vi "cam_wheel.vi"(7 "에러 입력":errorcluster, 10 "FPGA VI 참조 입력":refnum<k20>) -> (0 "에러 출력":errorcluster, 1 "거리":dbl, 2 "차체각도":dbl=-36.05, 3 "FPGA VI 참조 출력":refnum<k20>)   [LabVIEW 2019]
uses:
  <vilib>/Platform/TimedLoop/XDataNode/timing_clust.ctl
  <vilib>/Platform/TimedLoop/XDataNode/nitl_modes.ctl
  <vilib>/Platform/TimedLoop/XDataNode/wakeup.ctl
  <vilib>/myRIO/Instrument Drivers/Onboard IO/UART/typedef/VISA Configuration.ctl
  <vilib>/Utility/error.llb/Error Cluster From Error Code.vi
  <vilib>/rvi/errors/niLvFpgaAdjustHostInterfaceError.vi
  <vilib>/rvi/interface/nirviReadWriteControl/nirviReadWriteControl.xnode
  <vilib>/Platform/TimedLoop/XDataNode/XDataNode.xnode
  <vilib>/Platform/TimedLoop/XDataNode/XDNodeRunTimeDep.lvlib
  <vilib>/rvi/interface/Simulation/niFpgaSimulationCallBeginRW.vi
  NiFpgaLv.dll
  <vilib>/myRIO/Instrument Drivers/Onboard IO/UART/UART.lvlib
panel:
  out "pwm":dbl
  out "카메라 불인식 Y/N":bool
  in  "timed 정지":bool
  in  "Left":dbl[](array[numeric])=[2800.0, -379.347, 8600.0]
  in  "Right":dbl[](array[numeric])=[2800.0, 290.0, 8600.0]
  out "2번(불까지거리)":string
  out "1번(x픽셀)":string
  out "회전수 i":i32=148
  out "타임아웃":i32=-1
  out "L_encoder":i32
  out "R_Encoder":i32
  out "L_이동 거리":dbl=7.9770497222561305
  out "R_이동 거리":dbl=2.830566030477983
  out "mm/ms":dbl
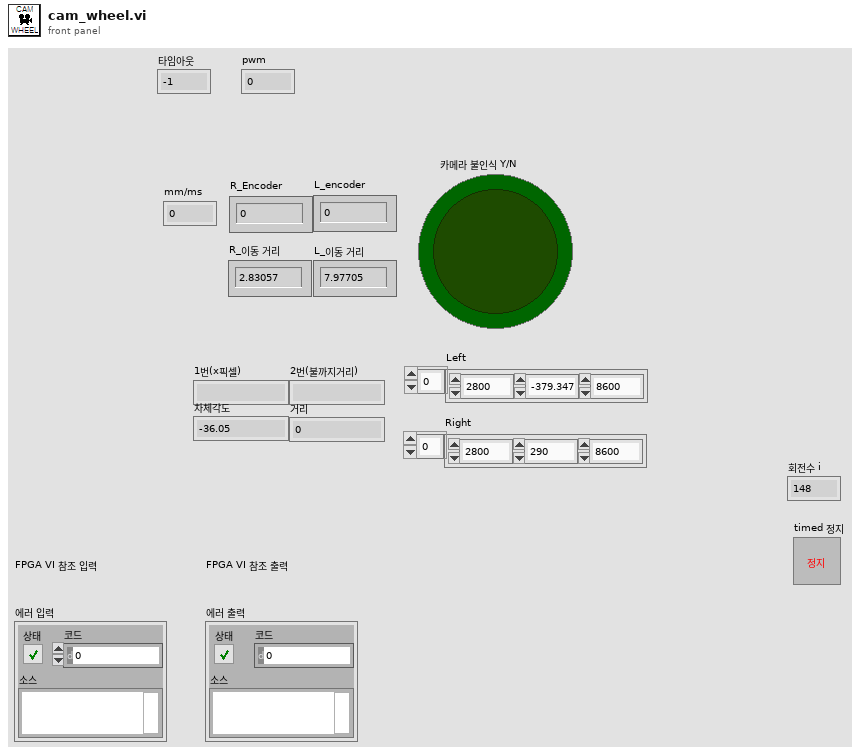
[diagram p1: front panel]
types:
  T1 = typedef "XDNodeRunTimeDep.lvlib/timing_clust.ctl" = cluster{"Expected End [f-1]":u64, "Actual End [f-1]":u64, "Finished Late? [f-1]":bool, "Expected End [i-1]":u64, "Actual End [i-1]":u64, "Finished Late? [i-1]":bool, "Expected Start [i]":u64, "Actual Start [i]":u64, "Expected Start [f]":u64, "Actual Start [f]":u64, "Source Name":string, "Structure Name":string, "Period":i64, "Deadline":i64, "Offset":i64, "Start":i64, "Priority":i32, "Timeout":i32, "Mode":T2, "Wakeup Reason":T3, "Error":errorcluster, "Source Type":string, "Secondary Source Type":string, "Global End Time":u64, "Global Start Time":u64, "Frame Duration":u64, "Iteration Duration":u64, "Assigned CPU":i32, "I/O Scan Engine Mode":u32}
  T2 = typedef "XDNodeRunTimeDep.lvlib/nitl_modes.ctl" = enum32{"No Change", "Process missed periods, maintain original phase", "Discard missed periods, maintain original phase", "Process missed periods, ignore original phase", "Discard missed periods, ignore original phase"}
  T3 = typedef "XDNodeRunTimeDep.lvlib/wakeup.ctl" = enum32{"Normal", "Aborted", "Asynchronous wakeup", "Timing source error", "Timed loop error", "Timeout"}
  T4 = typedef "UART.lvlib/VISA Configuration.ctl" = cluster{"baud rate (9600)":u32, "data bits (8)":u16, "parity (0:none)":enum16{"None", "Odd", "Even", "Mark", "Space"}, "stop bits (10: 1 bit)":u16, "flow control (0:none)":u16, "termination char\n(0xA = '\\n' = LF) ":u8, "Enable Termination\nChar (T)":bool, "timeout (10sec)":u32}
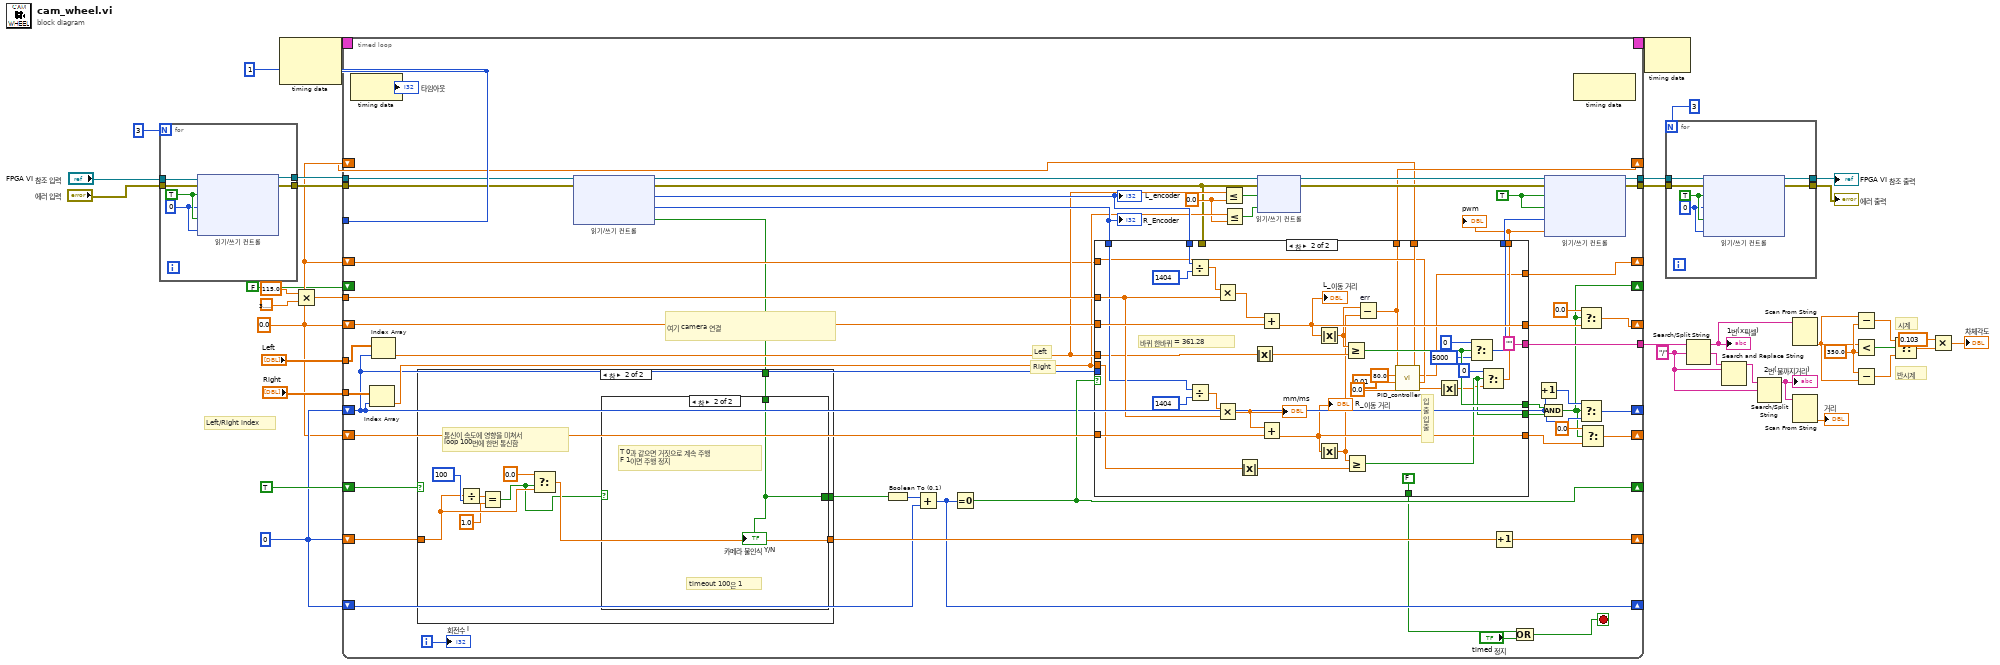
[diagram p0: block diagram]
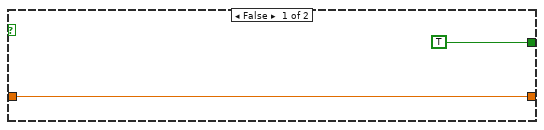
[diagram p2: hidden frame]
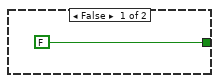
[diagram p3: hidden frame]
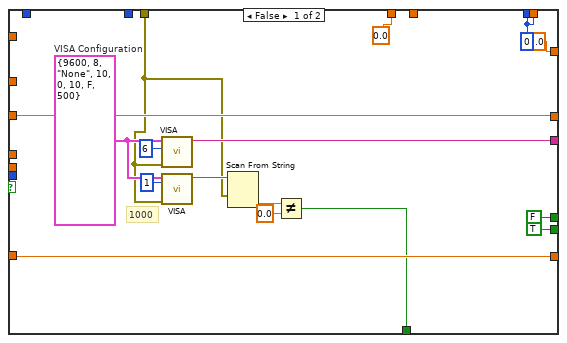
[diagram p4: hidden frame]
diagram:
  w10 = 350.0 ("y")
  w2 = 0.0
  w26 = "/" ("검색 문자열/문자 (-)")
  w14 = 0
  w28 = i64 1 ("주기")
  # "반시계"
  # "시계"
  # "Left/Right index"
  n1 = for {
    N: 3 -> [_]
    tunnel: [w43] -> w34
    tunnel: [w42] -> w33
    tunnel: "에러 입력" -> [w39]
    tunnel: "FPGA VI 참조 입력" -> [w38]
    w40 = 0 ("pwm input(escon)")
    w41 = TRUE ("encoder reset")
    n2 = xnode "읽기/쓰기 컨트롤"("FPGA VI 참조 입력"=w38, "에러 입력"=w39, "encoder reset"=w41, "pwm input"=w40, "R_encoder reset"=w41, "R_pwm input"=w40) -> ("FPGA VI 참조 출력"=w43:refnum<k20>, "에러 출력"=w42:errorcluster)
  }
  n3 = node-c288(w28) -> (w37:T1)  [unwired: 1 in]
  n4 = Multiply(x=115.0, y=3.141592653589793) -> (x*y=w29:dbl)
  n5 = timed-loop {
    timing: w37 -> [_]
    timing-out: [_] -> w36
    tunnel: w34 -> [w54]
    tunnel: w33 -> [w53]
    tunnel: [w97] -> w5
    tunnel: [w96] -> w4
    tunnel: w29 -> [w89]
    tunnel: w28 -> [_]
    shift-right: [w58] -> _
    shift-left: w2 -> [w90]
    shift-right: [w59] -> _
    shift-left: w2 -> [w91]
    shift-right: [w83] -> _
    shift-left: w14 -> [w81]
    shift-right: [w77] -> _
    shift-left: w14 -> [w78]
    shift-right: [w75] -> _
    shift-left: TRUE -> [w76]
    tunnel: [w74] -> w3
    tunnel: "Left" -> [w73]
    tunnel: "Right" -> [w72]
    shift-right: [w71] -> _
    shift-left: w14 -> [w51]
    shift-right: [w48] -> _
    shift-left: w2 -> [w45]
    shift-right: [w47] -> _
    shift-left: w2 -> [w46]
    shift-right: [w49] -> _
    shift-left: FALSE -> [_]
    i -> [w84]
    stop <- w60 stop-if-true
    w63 = 0.0 ("y")
    w95 = TRUE ("encoder reset")
    # "여기 camera 연결"
    # "Right"
    # "Left"
    n6 = node-c288() -> (→"타임아웃":i32)  [unwired: 1 in]
    n7 = Index Array(array=w72, index=w51) -> (element=w66:dbl)
    n8 = Index Array(array=w73, index=w51) -> (element=w67:dbl)
    n9 = xnode "읽기/쓰기 컨트롤"("FPGA VI 참조 입력"=w54, "에러 입력"=w53) -> ("FPGA VI 참조 출력"=w93:refnum<k20>, "에러 출력"=w52:errorcluster, "Encoder  (4x)"=w88:i32, "R_Encoder  (4x)"=w87:i32, "camera"=w44:bool)
    "L_encoder" <- w88
    "R_Encoder" <- w87
    n10 = case shown="참" w76 {
      tunnel: [w99 w108] -> w82
      tunnel: w81 -> [w99 w106]
      tunnel: [TRUE w102] -> w79
      tunnel: w44 -> [_ w101]
      frame False {
      }
      frame True {
        # "통신이 속도에 영향을 미쳐서\nloop 100번에 한번 통신함"
        n11 = Divide(x=w106, y=100) -> (x/y=w105:dbl)
        n12 = Equal?(x=w105, y=1.0) -> (x = y?=w103:bool)
        n13 = Select(t=0.0, s=w103, f=w106) -> (s? t:f=w108:dbl)
        n14 = case shown="참" w103 {
          tunnel: [FALSE w111] -> w102
          tunnel: w101 -> [_ w111]
          frame False {
          }
          frame True {
            # "timeout 100은 1"
            # "T 0과 같으면 거짓으로 계속 주행\nF 1이면 주행 정지"
            "카메라 불인식 Y/N" <- w111
          }
        }
      }
    }
    n15 = Boolean To (0,1)(Boolean=w79) -> (0, 1=w80:i16)
    n16 = Add(x=w80, y=w78) -> (x+y=w77:i32)
    n17 = Equal To 0?(x=w77) -> (x = 0?=w75:bool)
    n18 = case shown="참" w75 {
      tunnel: [w125 w164] -> w55
      tunnel: w91 -> [w126 w163]
      tunnel: w90 -> [w125 w162]
      tunnel: w89 -> [_ w161]
      tunnel: w88 -> [_ w160]
      tunnel: w87 -> [_ w159]
      tunnel: [w118 FALSE] -> w62
      tunnel: [w127 w152] -> w86
      tunnel: [w127 w149] -> w85
      tunnel: [w126 w148] -> w56
      tunnel: [w123 "" ("read buffer")] -> w74
      tunnel: w67 -> [_ w142]
      tunnel: w66 -> [_ w140]
      tunnel: [FALSE w145] -> w69
      tunnel: [TRUE w144] -> w68
      tunnel: w52 -> [w114 _]
      tunnel: w51 -> [_ _]
      tunnel: w45 -> [_ w135]
      tunnel: [0.0 w128] -> w48
      tunnel: w46 -> [_ w132]
      tunnel: [0.0 ("Error_Sum(k)") w131] -> w47
      frame False {
        w117 = T4 {"baud rate (9600)"=9600, "data bits (8)"=8, "parity (0:none)"=enum."None", "stop bits (10: 1 bit)"=10, "flow control (0:none)"=0, "termination char\n(0xA = '\\n' = LF) "=10, "Enable Termination\nChar (T)"=FALSE, "timeout (10sec)"=500}  # VISA Configuration
        w127 = 0 ("L_pwm")
        # "1000"
        n19 = call "VISA.vi"("에러 입력(에러 없음)"=w114, "바이트 카운트"=u32 6, "VISA Configuration"=w117) -> ("read buffer"=w123:string)  [unwired: 7 in, 1 out]
        n20 = call "VISA.vi"("에러 입력(에러 없음)"=w114, "바이트 카운트"=u32 1, "VISA Configuration"=w117) -> ("read buffer"=w116:string)  [unwired: 7 in, 1 out]
        n21 = Scan From String(input string=w116, error in=w114) -> (output 1=w120:dbl)  [unwired: 3 in, 3 out]
        n22 = Not Equal?(x=w120, y=0.0) -> (x != y?=w118:bool)
      }
      frame True {
        # "입\n출\n입\n출"
        # "바퀴 한바퀴 = 361.28"
        n23 = Divide(x=w160, y=1404) -> (x/y=w156:dbl)
        n24 = Divide(x=w159, y=1404) -> (x/y=w153:dbl)
        n25 = Multiply(x=w156, y=w161) -> (x*y=w157:dbl)
        n26 = Multiply(x=w153, y=w161) -> (x*y=w154:dbl)
        "mm/ms" <- w154
        n27 = Absolute Value(x=w140) -> (abs(x)=w141:dbl)
        n28 = Absolute Value(x=w142) -> (abs(x)=w143:dbl)
        n29 = Add(x=w157, y=w162) -> (x+y=w164:dbl)
        "L_이동 거리" <- w164
        n30 = Add(x=w154, y=w163) -> (x+y=w148:dbl)
        "R_이동 거리" <- w148
        n31 = Absolute Value(x=w164) -> (abs(x)=w134:dbl)
        n32 = Absolute Value(x=w148) -> (abs(x)=w133:dbl)
        n33 = Greater Or Equal?(x=w134, y=w143) -> (x >= y?=w145:bool)
        n34 = Greater Or Equal?(x=w133, y=w141) -> (x >= y?=w144:bool)
        n35 = Subtract "err"(x=w134, y=w133) -> (x-y=w128:dbl)
        n36 = call "PID_controller.vi"("Error_Sum(k-1)"=w132, "Error(k-1)"=w135, "Ki"=0.0, "Kd"=0.01, "Kp"=80.0, "Error(k)"=w128) -> ("u(k)"=w130:dbl, "Error_Sum(k)"=w131:dbl)
        n37 = Absolute Value(x=w130) -> (abs(x)=w129:dbl)
        n38 = Select(t=0, s=w145, f=5000) -> (s? t:f=w152:i32)
        n39 = Select(t=0, s=w144, f=w129) -> (s? t:f=w149:dbl)
      }
    }
    "pwm" <- w85
    n40 = Less Or Equal?(x=w67, y=w63) -> (x <= y?=w65:bool)
    n41 = Less Or Equal?(x=w66, y=w63) -> (x <= y?=w64:bool)
    n42 = xnode "읽기/쓰기 컨트롤"("FPGA VI 참조 입력"=w93, "에러 입력"=w52, "L_dir"=w65, "R_dir"=w64) -> ("FPGA VI 참조 출력"=w94:refnum<k20>, "에러 출력"=w92:errorcluster)
    n43 = Increment(x=w82) -> (x+1=w83:dbl)
    n44 = Or(x=w62, y="timed 정지") -> (x .or. y?=w60:bool)
    n45 = Increment(x=w51) -> (x+1=w70:i32)
    n46 = And(x=w69, y=w68) -> (x .and. y?=w49:bool)
    n47 = xnode "읽기/쓰기 컨트롤"("FPGA VI 참조 입력"=w94, "에러 입력"=w92, "encoder reset"=w95, "R_encoder reset"=w95, "pwm input"=w86, "R_pwm input"=w85) -> ("FPGA VI 참조 출력"=w97:refnum<k20>, "에러 출력"=w96:errorcluster)
    n48 = node-c288() -> ()  [unwired: 1 in, 1 out]
    n49 = Select(t=0.0, s=w49, f=w55) -> (s? t:f=w58:dbl)
    n50 = Select(t=w70, s=w49, f=w51) -> (s? t:f=w71:i32)
    n51 = Select(t=0.0, s=w49, f=w56) -> (s? t:f=w59:dbl)
    "회전수 i" <- w84
  }
  n52 = node-c288(w36) -> ()  [unwired: 1 out]
  n53 = for {
    N: 3 -> [_]
    tunnel: [w171] -> w21
    tunnel: [w170] -> w20
    tunnel: w5 -> [w169]
    tunnel: w4 -> [w168]
    w172 = 0 ("pwm input(escon)")
    w173 = TRUE ("encoder reset")
    n54 = xnode "읽기/쓰기 컨트롤"("FPGA VI 참조 입력"=w169, "에러 입력"=w168, "encoder reset"=w173, "pwm input"=w172, "R_encoder reset"=w173, "R_pwm input"=w172) -> ("FPGA VI 참조 출력"=w171:refnum<k20>, "에러 출력"=w170:errorcluster)
  }
  "FPGA VI 참조 출력" <- w21
  "에러 출력" <- w20
  n55 = Search/Split String(string=w3, search string/char (-)=w26) -> (substring before match=w19:string, match + rest of string=w25:string)  [unwired: 2 out]
  "1번(x픽셀)" <- w19
  n56 = Search and Replace String(input string=w25, search string=w26) -> (result string=w24:string)  [unwired: 1 in, 8 out]
  n57 = Search/Split String(string=w24, search string/char (-)=w26) -> (substring before match=w18:string)  [unwired: 3 out]
  "2번(불까지거리)" <- w18
  n58 = Scan From String(input string=w19) -> (output 1=w9:dbl)  [unwired: 4 in, 3 out]
  n59 = Scan From String(input string=w18) -> (output 1=→"거리":dbl)  [unwired: 4 in, 3 out]
  n60 = Subtract(x=w9, y=w10) -> (x-y=w12:dbl)
  n61 = Less?(x=w9, y=w10) -> (x < y?=w13:bool)
  n62 = Subtract(x=w10, y=w9) -> (x-y=w11:dbl)
  n63 = Select(t=w12, s=w13, f=w11) -> (s? t:f=w8:dbl)
  n64 = Multiply(x=0.103, y=w8) -> (x*y=→"차체각도":dbl)
